vi "IO_ClassTypeData.vi"() -> ()   [LabVIEW 2019]
uses:
  IO_Class/IOCard.lvclass
panel:
  in  "IOQue":refnum<queue>[](array[refnum])
  out "IOCard":refnum<class "IOCard.lvclass">[](array[class])
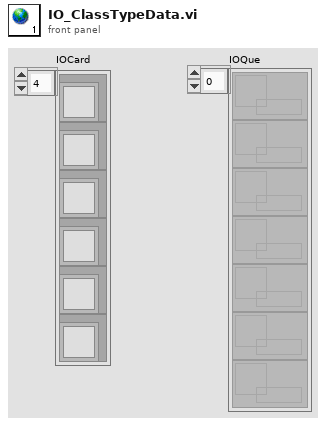
[diagram p1: front panel]
diagram:
